vi "Dashboard Main.vi"() -> ()   [LabVIEW 2012]
uses:
  <vilib>/event_ctls.llb/eventvkey.ctl
  <vilib>/Rock Robotics/Network Tables/NT Read Name Cache.vi
  <vilib>/Rock Robotics/Network Tables/NT Globals.vi
  <vilib>/Rock Robotics/Network Tables/Field Data Manager.vi
  <vilib>/Rock Robotics/Network Tables/Table Manager.vi
  <vilib>/Rock Robotics/Network Tables/Report Read Error.vi
panel:
  out "Mode":enum8{"Tele-Op", "Auto", "Test", ""}(ring)=enum."Test"
  out "Camera IP":string
  out "JS1 Z":dbl(slide) scale=-1.0..1.0 scale format="%#_2e"
  out "JS2 Z":dbl(slide) scale=-1.0..1.0 scale format="%#_2e"
  out "Joystick 1":cluster{"X":dbl, "Y":dbl}[](graph)
  out "Joystick 2":cluster{"X":dbl, "Y":dbl}[](graph)
  out "JS Buttons 1":T1
  out "JS Buttons 2":T1
  out "MotorSlide4":dbl(slide) scale=-1.0..1.0 scale format="%#_2e"
  out "MotorSlide3":dbl(slide) scale=-1.0..1.0 scale format="%#_2e"
  out "MotorSlide2":dbl(slide) scale=-1.0..1.0 scale format="%#_2e"
  in  "MotorName3":string="Front Left"
  in  "MotorName4":string="Front Right"
  in  "MotorName1":string="Rear Left"
  in  "MotorName2":string="Rear Right"
  out "MotorChart4":dbl(graph)
  out "MotorChart3":dbl(graph)
  out "MotorChart2":dbl(graph)
  out "MotorSlide1":dbl(slide) scale=-1.0..1.0 scale format="%#_2e"
  out "MotorChart1":dbl(graph)
  out "Battery Value":dbl(slide) scale=0.0..14.0 scale format="%#_2e"
  out "Robot IP":string
  out "Battery":sgl(graph)
  in  "Dashboard Tab":enum32{"Operation", "Test", "Checklist"}(tab)
  out "Motor 0":dbl
  out "Motor 4":dbl
  out "Motor 3":dbl
  out "Motor 2":dbl
  out "Motor 1":dbl
  out "Y Axis":dbl
  out "X Axis":dbl
  in  "Checkbox 2":bool
  in  "Checkbox 1":bool
  in  "Slider 1":dbl(slide) scale=0.0..100.0
  in  "ServoValue":dbl(slide) scale=0.0..170.0 scale format="%#_3g"
  in  "On/Off":bool caption="Solenoid"
  in  "Test Name":u16(ring) items=["Select the test to run...", "Example Test", "", "Tests are read from", "Public\\Documents\\FRC\\Tests.txt", "", "Modify file to customize list."]
  in  "Test Tree":string(tree)
  in  "Motor":cluster{"Value":dbl, "Enable":bool} {"Value" scale=-1.0..1.0 scale format="%#_3g"}
  out "Progress":T2 {"Test Progress" scale=0.0..100.0}
  in  "Rev/Fwd":cluster{"Forward":bool, "Reverse":bool}
  in  "Listbox":i32(listbox)
  in  "Viewer":T3(tab)
  out "Image Error Message":string="Timeout in Camera Communications"
  in  "Video Enable":bool=TRUE
  out "Camera Image":T4(plugin-control)
  out "Buttons 1":cluster{"1":bool, "2":bool, "3":bool}
  out "Kinect 1":cluster{"X":dbl, "Y":dbl, "Z":dbl} {"X" scale=1.0..-1.0; "Y" scale=1.0..-1.0; "Z" scale=1.0..-1.0}
  out "Buttons 2":cluster{"1":bool, "2":bool, "3":bool}
  out "Kinect 2":cluster{"X":dbl, "Y":dbl, "Z":dbl} {"X" scale=1.0..-1.0; "Y" scale=1.0..-1.0; "Z" scale=1.0..-1.0}
  out "Version":string
  out "Skeleton Picture":picture
  out "Players":i8
  out "Tree":string(tree)
  # "Drive & Motors"
  # "Robot IP:"
  # "Customize by placing controls and indicators here and name to match\nDashboard Variables on robot."
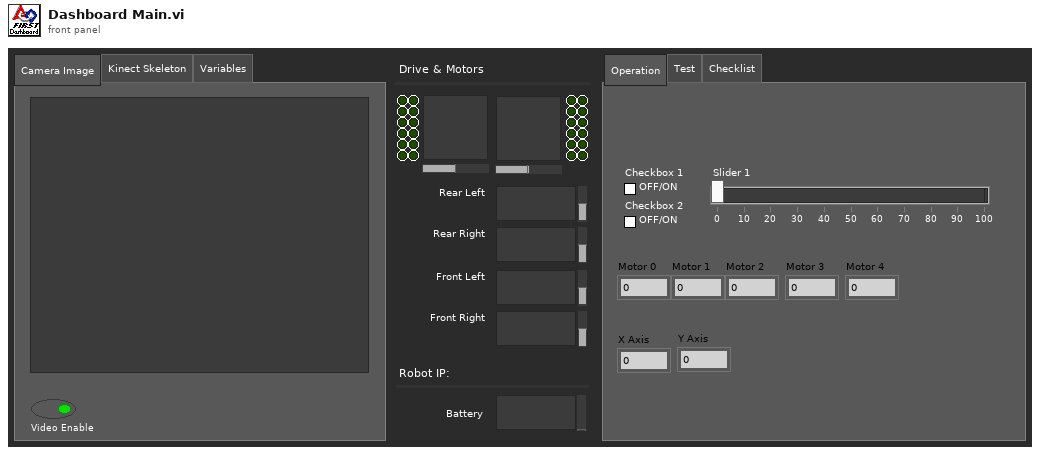
[diagram p1: front panel]
types:
  T1 = cluster{bool, bool, bool, bool, bool, bool, bool, bool, bool, bool, bool, bool}
  T2 = cluster{"Test Progress":u8, "Test Progress Text":string}
  T3 = enum32{"Camera Image", "Kinect Skeleton", "Variables"}
  T4 = typedef "IMAQ Image.ctl" = refnum<image>
  T5 = typedef "Image Type" = u32
  T6 = typedef "SkeletonTrackState.ctl" = enum32{"NotTracked", "PositionOnly", "Tracked"}
  T7 = cluster{"TrackingState":u8[], "Position":cluster{"x":sgl, "y":sgl, "z":sgl}, cluster{"x":sgl, "y":sgl, "z":sgl, sgl}[], "TrackState":T6}
  T8 = cluster{cluster{"ScaledToPercentRange":dbl, "ScaledToPercentRange":dbl, "ScaledToPercentRange":dbl}, cluster{bool, bool, bool}}[]
  T9 = typedef "LVBoundsTypeDef.ctl" = cluster{"Width":u32, "Height":u32}
  T10 = cluster{cluster{"ScaledToPercentRange":dbl, "ScaledToPercentRange":dbl, "ScaledToPercentRange":dbl}, cluster{bool, bool, bool}}
  T11 = cluster{"ScaledToPercentRange":dbl, "ScaledToPercentRange":dbl, "ScaledToPercentRange":dbl}
  T12 = typedef "LVRectTypeDef.ctl" = cluster{"Left":i16, "Top":i16, "Right":i16, "Bottom":i16}
  T13 = cluster{"Competition mode":bool, "Robot Link":bool, "Autonomous":bool, "Enabled":bool, "E-Stop":bool, "Simulated":bool, "TestMode":bool, "Docked Window":bool}
  T14 = cluster{"Boolean Array[0]":bool, "Boolean Array[1]":bool, "Boolean Array[2]":bool, "Boolean Array[3]":bool, "Boolean Array[4]":bool, "Boolean Array[5]":bool, "Boolean Array[6]":bool, "Boolean Array[7]":bool, "Boolean Array[8]":bool, "Boolean Array[9]":bool, "Boolean Array[10]":bool, "Boolean Array[11]":bool}
  T15 = typedef "eventvkey.ctl" = enum16{"ASCII", "Enter", "Return", "Shift", "Ctrl", "Alt", "Cmd", "Opt", "Caps", "NumLock", "Clear", "Break", "Up", "Down", "Left", "Right", "Insert", "Delete", "Home", "End", "PageUp", "PageDown", "Escape", "Help", "Pause", "ScrollLock", "F1", "F2", "F3", "F4", "F5", "F6", "F7", "F8", "F9", "F10", "F11", "F12", "F13", "F14", "F15", "F16", "F17", "F18", "F19", "F20", "F21", "F22", "F23", "F24", "Play", "VolumeUp", "VolumeDown", "Mute", "Two Byte Char"}
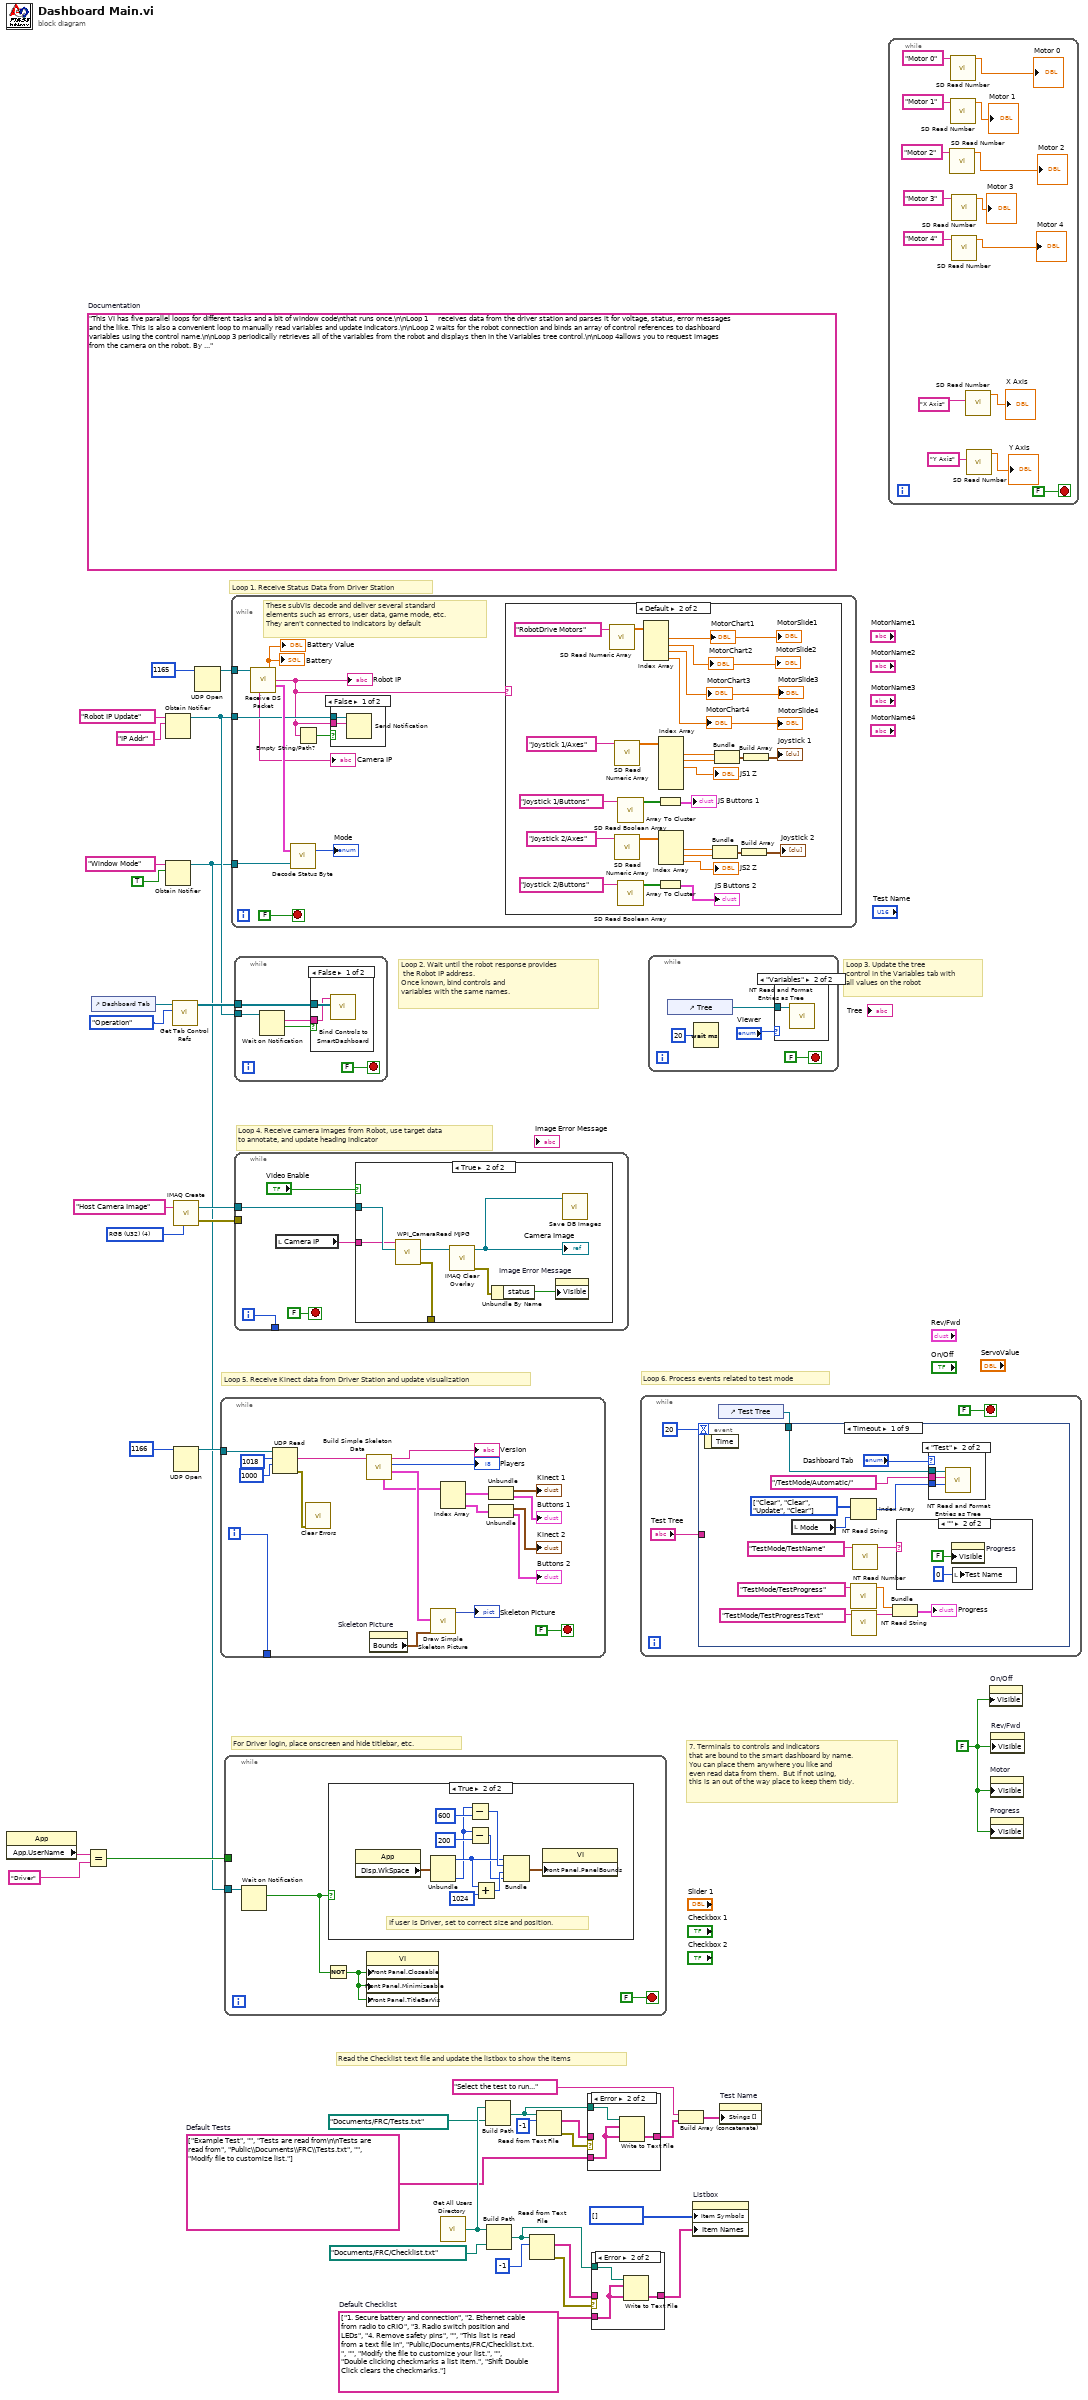
[diagram p0: block diagram]
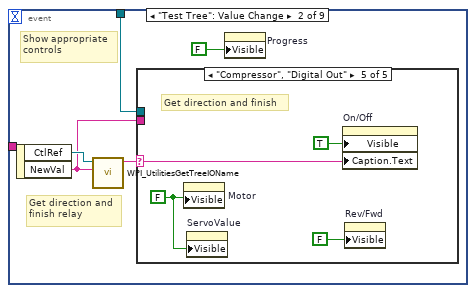
[diagram p7: hidden frame]
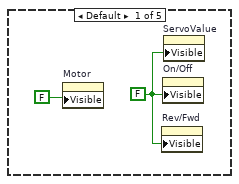
[diagram p8: hidden frame]
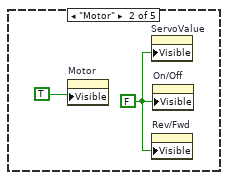
[diagram p9: hidden frame]
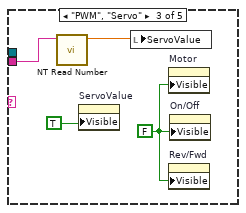
[diagram p10: hidden frame]
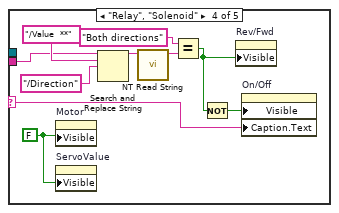
[diagram p11: hidden frame]
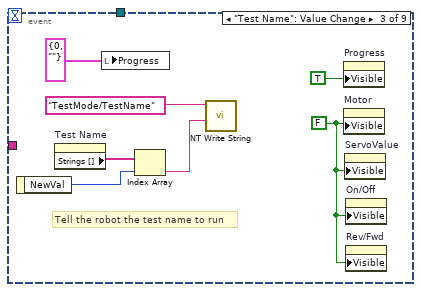
[diagram p12: hidden frame]
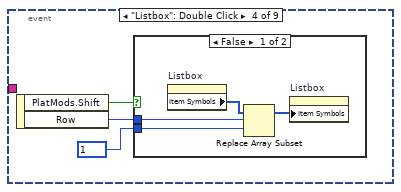
[diagram p13: hidden frame]
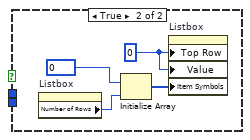
[diagram p14: hidden frame]
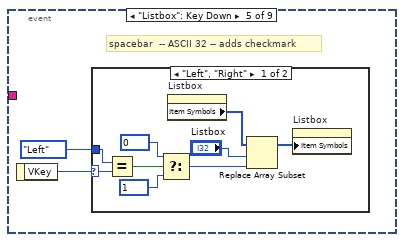
[diagram p15: hidden frame]
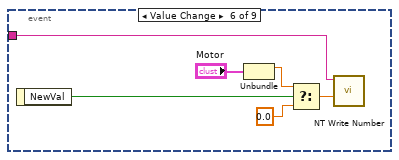
[diagram p17: hidden frame]
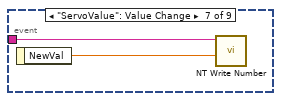
[diagram p18: hidden frame]
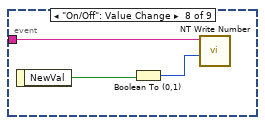
[diagram p19: hidden frame]
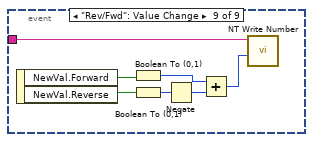
[diagram p20: hidden frame]
diagram:
  w3 = string[] ["1. Secure battery and connection", "2. Ethernet cable from radio to cRIO", "3. Radio switch position and LEDs", "4. Remove safety pins", "", "This list is read from a text file in", "Public/Documents/FRC/Checklist.txt.", "", "Modify the file to customize your list.", "", "Double clicking checkmarks a list item.", "Shift Double Click clears the checkmarks."]  # Default Checklist
  w8 = string[] ["Example Test", "", "Tests are read from\n\nTests are read from", "Public\\Documents\\FRC\\Tests.txt", "", "Modify file to customize list."]  # Default Tests
  w1 = FALSE ("Visible")
  (unwired) "This VI has five parallel loops for different tasks and a bit of window code\nthat runs once.\n\nLoop 1     receives data from the driver station and parses it for voltage, status, error messages and the like. This is also a convenient loop to manually read variables and update indicators.\n\nLoop 2 waits for the robot connection and binds an array of control references to dashboard variables using the control name.\n\nLoop 3 periodically retrieves all of the variables from the robot and displays then in the Variables tree control.\n\nLoop 4allows you to request images from the camera on the robot. By default, it reads the images using MJPG stream, but has compatibility for the older setup which used JPGs.\n\nLoop 5 processes any data from the Kinect server and shows the skeleton and Kinect stick values in the Kinect tab.\n\nLoop 6 process events for the TestMode tree, listbox, ring, and actuator\n\nLoop 7 calculates and updates the window location, size, and style. The checklist and tests are loaded from text files and placed into the controls.\n\nAdding new indicators or controls:\nAdd them to the panel in the Operations tab and name them the same as the SmartDashboard variable on the robot. The binding loop will keep them synchronized."  # Documentation
  w37 = T5 4 items=["Grayscale (U8)", "Grayscale (I16)", "Grayscale (SGL)", "Complex (CSG)", "RGB (U32)", "HSL (U32)", "RGB (U64)"] ("Image Type")
  # "Loop 6. Process events related to test mode"
  # "Read the Checklist text file and update the listbox to show the items"
  # "7. Terminals to controls and indicators\nthat are bound to the smart dashboard by name.\nYou can place them anywhere you like and\neven read data from them.  But if not using,\nthis is an out of the way place to keep them tidy."
  # "Loop 3. Update the tree\ncontrol in the Variables tab with\nall values on the robot"
  # "Loop 2. Wait until the robot response provides\n the Robot IP address.\nOnce known, bind controls and\nvariables with the same names."
  # "Loop 5. Receive Kinect data from Driver Station and update visualization"
  # "For Driver login, place onscreen and hide titlebar, etc."
  # "Loop 1. Receive Status Data from Driver Station"
  # "Loop 4. Receive camera images from Robot, use target data\nto annotate, and update heading indicator"
  n1 = property class="App"() -> ("App.UserName"=w32:string)  [unwired: 2 in, 2 out]
  n2 = Equal?(x=w32, y="Driver") -> (x = y?=w31:bool)
  n3 = control-ref of="Dashboard Tab"() -> (w27:refnum<vi>)
  n4 = Obtain Notifier(name (unnamed)="Robot IP Update", notification data type="IP Addr" ("name (unnamed)")) -> (notifier out=w24:refnum<notifier>)  [unwired: 2 in, 2 out]
  n5 = Obtain Notifier(name (unnamed)="Window Mode", notification data type=TRUE) -> (notifier out=w12:refnum<notifier>)  [unwired: 2 in, 2 out]
  n6 = call <vilib>:"Get Tab Control Refs.vi"("Page Index"=enum32{"Operation", "Test"}."Operation" ("Dashboard Tab"), "TabControl in"=w27) -> ("ControlsOnPage"=w28:refnum<vi>[])  [unwired: 9 in]
  n7 = call "IMAQ Create"("Image Name"="Host Camera Image", "Image Type"=w37) -> ("New Image"=w35:T4, "error out"=w34:errorcluster)  [unwired: 2 in, 1 out]
  n8 = UDP Open(11:u16 1166 ("port")) -> (port=w29:refnum<k16>)  [unwired: 2 in, 4 out]
  n9 = UDP Open(11:u16 1165 ("port")) -> (port=w38:refnum<k16>)  [unwired: 2 in, 4 out]
  n10 = while {
    tunnel: w29 -> [w56]
    tunnel: [w40] -> _
    i -> [w40]
    stop <- FALSE stop-if-true
    n11 = UDP Read(connection ID=w56, max size (548)=1018 ("bytes to read"), timeout ms (25000)=1000) -> (data out=w50:string, error out=w48:errorcluster)  [unwired: 1 in, 3 out]
    n12 = call <vilib>:"Clear Errors.vi"("error in (no error)"=w48) -> ()  [unwired: 6 in, 1 out]
    n13 = call "Build Simple Skeleton Data.vi"("data out"=w50) -> ("Skeleton Data"=w51:T7, "NumPlayers"=→"Players":i8, "Version String"=→"Version":string, "Simple Joystick Info"=w47:T8)  [unwired: 6 in, 1 out]
    n14 = property on="Skeleton Picture" class="Pict"() -> ("Bounds"=w52:T9)  [unwired: 2 in, 2 out]
    n15 = call "Draw Simple Skeleton Picture.vi"("Bounds"=w52, "Simple Skeleton"=w51) -> ("new picture out"=→"Skeleton Picture":picture)  [unwired: 9 in]
    n16 = Index Array(array=w47) -> (element #1=w46:T10, element #2=w45:T10)  [unwired: 2 in]
    n17 = Unbundle(w46) -> (→"Kinect 1":T11, →"Buttons 1":cluster{bool, bool, bool})
    n18 = Unbundle(w45) -> (→"Kinect 2":T11, →"Buttons 2":cluster{bool, bool, bool})
  }
  n19 = while {
    tunnel: w31 -> [_]
    tunnel: w12 -> [w61]
    stop <- FALSE stop-if-true
    n20 = Wait on Notification(notifier=w61) -> (notification=w59:bool)  [unwired: 3 in, 3 out]
    n21 = Not(x=w59) -> (.not. x?=w60:bool)
    n22 = case shown="True" w59 {
      frame False {
      }
      frame True {
        # "If user is Driver, set to correct size and position."
        n23 = property class="App"() -> ("Disp.WkSpace"=w72:T12)  [unwired: 2 in, 2 out]
        n24 = Unbundle(w72) -> ("Left"=w67:i16, "Bottom"=w63:i16)  [unwired: 2 out]
        n25 = Subtract(x=w63, y=600) -> (x-y=w69:i32)
        n26 = Subtract(x=w63, y=200) -> (x-y=w64:i32)
        n27 = Add(x=w67, y=1024) -> (x+y=w68:i32)
        n28 = Bundle("Left"=w67, w69, w68, w64) -> (w71:cluster{"Left":i16, i32, i32, i32})  [unwired: 1 out]
        n29 = property class="VI"("Front Panel.PanelBounds"=w71) -> ()  [unwired: 2 in, 2 out]
      }
    }
    n30 = property class="VI"("Front Panel.Closeable"=w60, "Front Panel.Minimizeable"=w60, "Front Panel.TitleBarVis"=w60) -> ()  [unwired: 2 in, 2 out]
  }
  n31 = while {
    tunnel: w38 -> [w80]
    tunnel: w24 -> [w78]
    tunnel: w12 -> [w75]
    stop <- FALSE stop-if-true
    # "These subVIs decode and deliver several standard\nelements such as errors, user data, game mode, etc.\nThey aren't connected to indicators by default"
    n32 = call "Receive DS Packet.vi"("Recv Socket"=w80) -> ("Battery"=→"Battery" →"Battery Value":sgl, "Robot IP Address"=w77:string, "Status"=w81:T13, "Camera IP Address"=→"Camera IP":string)  [unwired: 1 in, 10 out]
    "Robot IP" <- w77
    n33 = call "Decode Status Byte.vi"("Window Mode Notifier"=w75, "Status"=w81) -> ("Mode"=→"Mode":enum8{"Tele-Op", "Auto", "Test", ""})  [unwired: 1 out]
    n34 = Empty String/Path?(string/path=w77) -> (empty?=w76:bool)
    n35 = case shown="False" w76 {
      tunnel: w78 -> [w110 _]
      tunnel: w77 -> [w109 _]
      frame False {
        n36 = Send Notification(notification=w109, notifier=w110) -> ()  [unwired: 1 in, 2 out]
      }
      frame True {
      }
    }
    n37 = case shown="Default" w77 {
      frame "" {
        # "Robot not responding, don't poll the variables"
      }
      frame Default {
        n38 = call <vilib>:"SD Read Numeric Array.vi"("Name"="RobotDrive Motors") -> ("Numeric Array"=w105:dbl[])  [unwired: 8 in, 2 out]
        n39 = call <vilib>:"SD Read Numeric Array.vi"("Name"="Joystick 1/Axes") -> ("Numeric Array"=w98:dbl[])  [unwired: 8 in, 2 out]
        n40 = call <vilib>:"SD Read Numeric Array.vi"("Name"="Joystick 2/Axes") -> ("Numeric Array"=w92:dbl[])  [unwired: 8 in, 2 out]
        n41 = call <vilib>:"SD Read Boolean Array.vi"("Name"="Joystick 1/Buttons") -> ("Boolean Array"=w100:bool[])  [unwired: 8 in, 2 out]
        n42 = call <vilib>:"SD Read Boolean Array.vi"("Name"="Joystick 2/Buttons") -> ("Boolean Array"=w91:bool[])  [unwired: 8 in, 2 out]
        n43 = Index Array(array=w105) -> (element #1=→"MotorChart1" →"MotorSlide1":dbl, element #2=→"MotorSlide2" →"MotorChart2":dbl, element #3=→"MotorChart3" →"MotorSlide3":dbl, element #4=→"MotorChart4" →"MotorSlide4":dbl)  [unwired: 4 in]
        n44 = Array To Cluster(array=w100) -> (cluster=→"JS Buttons 1":T14)
        n45 = Array To Cluster(array=w91) -> (cluster=→"JS Buttons 2":T14)
        n46 = Index Array(array=w98) -> (element #1=w95:dbl, element #2=w96:dbl, element #3=→"JS1 Z":dbl)  [unwired: 6 in, 3 out]
        n47 = Index Array(array=w92) -> (element #1=w87:dbl, element #2=w86:dbl, element #3=→"JS2 Z":dbl)  [unwired: 3 in]
        n48 = Bundle("Numeric"=w87, "Numeric"=w86) -> (w88:cluster{"Numeric":dbl, "Numeric":dbl})  [unwired: 1 in]
        n49 = Bundle("Numeric"=w95, "Numeric"=w96) -> (w94:cluster{"Numeric":dbl, "Numeric":dbl})  [unwired: 1 in]
        n50 = Build Array(w88) -> (→"Joystick 2":cluster{"Numeric":dbl, "Numeric":dbl}[])
        n51 = Build Array(w94) -> (→"Joystick 1":cluster{"Numeric":dbl, "Numeric":dbl}[])
      }
    }
  }
  n52 = while {
    tunnel: w28 -> [w115]
    tunnel: w24 -> [w112]
    stop <- FALSE stop-if-true
    n53 = Wait on Notification(notifier=w112) -> (notification=w111:string, timed out?=w113:bool)  [unwired: 3 in, 2 out]
    n54 = case shown="False" w113 {
      tunnel: w115 -> [w117 _]
      tunnel: w111 -> [w116 _]
      frame False {
        n55 = call <vilib>:"Bind Controls to SmartDashboard.vi"("Bound Control Refs"=w117, "Server IP Address"=w116) -> ()  [unwired: 10 in]
      }
      frame True {
      }
    }
  }
  n56 = while {
    tunnel: w35 -> [w121]
    tunnel: w34 -> [_]
    tunnel: [w119] -> _
    i -> [w119]
    stop <- FALSE stop-if-true
    n57 = local read "Camera IP"() -> (w118:string)
    n58 = case shown="True" "Video Enable" {
      tunnel: w118 -> [w125 w127]
      tunnel: w121 -> [w124 w133]
      tunnel: [_ w128] -> _
      frame False {
        # "Sleep for 500ms"
        n59 = call <vilib>:"WPI_CameraRead MJPG.vi"("Operation"=enum16{"Read", "Reopen", "Close"}."Close", "Image"=w124, "address"=w125) -> ()  [unwired: 7 in, 2 out]
        n60 = Wait Until Next ms Multiple(millisecond multiple=u32 500) -> ()  [unwired: 1 out]
      }
      frame True {
        n61 = call <vilib>:"WPI_CameraRead MJPG.vi"("Image"=w133, "address"=w127) -> ("error out"=w128:errorcluster, "Image Out"=w130:T4)  [unwired: 8 in]
        n62 = call "IMAQ Clear Overlay"("Image"=w130) -> ("error out"=w131:errorcluster, "Image Out"=w129:T4)  [unwired: 2 in, 7 out]
        "Camera Image" <- w129
        n63 = Unbundle By Name(w131) -> ("status"=w132:bool)
        n64 = property on="Image Error Message" class="Str"("Visible"=w132) -> ()  [unwired: 2 in, 2 out]
        n65 = call "Save DB Images.vi"("Image"=w129) -> ()  [unwired: 2 in, 1 out]
      }
    }
  }
  n66 = call "Get All Users Directory.vi"() -> ("All User Path"=w19:path)
  n67 = Build Path(base path=w19, name or relative path=path "Documents/FRC/Tests.txt") -> (appended path=w7:path)
  n68 = Build Path(base path=w19, name or relative path=path "Documents/FRC/Checklist.txt") -> (appended path=w4:path)
  n69 = Read from Text File(file (use dialog)=w4, count=-1 ("timeout ms (25000)")) -> (text=w5:string[], error out=w6:errorcluster)  [unwired: 2 in, 2 out]
  n70 = Read from Text File(file (use dialog)=w7, count=-1 ("timeout ms (25000)")) -> (text=w10:string[], error out=w11:errorcluster)  [unwired: 2 in, 2 out]
  n71 = case shown="Error" w11 {
    tunnel: w10 -> [w134 _]
    tunnel: [w134 w135] -> w9
    tunnel: w8 -> [_ w135]
    tunnel: w7 -> [_ w136]
    frame No Error {
    }
    frame Error {
      n72 = Write to Text File(file (use dialog)=w136, text=w135) -> ()  [unwired: 2 in, 3 out]
    }
  }
  n73 = case shown="Error" w6 {
    tunnel: w5 -> [w137 _]
    tunnel: [w137 w138] -> w2
    tunnel: w3 -> [_ w138]
    tunnel: w4 -> [_ w139]
    frame No Error {
    }
    frame Error {
      n74 = Write to Text File(file (use dialog)=w139, text=w138) -> ()  [unwired: 2 in, 3 out]
    }
  }
  n75 = while {
    stop <- FALSE stop-if-true
    n76 = control-ref of="Test Tree"() -> (w141:refnum<vi>)
    n77 = event shown="[0] Timeout" {
      selector: _ -> [_ _ _ _ _ _ _ _ _]
      dyn-events: _ -> [_ _ _ _ _ _ _ _ _]
      timeout: u32 20 ("milliseconds to wait") -> [_ _ _ _ _ _ _ _ _]
      tunnel: w141 -> [w152 w163 _ _ _ _ _ _ _]
      tunnel: "Test Tree" -> [_ _ _ _ _ w218 w225 w226 w229]
      event Timeout {
        w145 = enum16{"Update", "Clear"}[] [enum."Clear", enum."Clear", enum."Update", enum."Clear"] items=["Update", "Clear"]
        n78 = event-data() -> ()  [unwired: 1 in, 1 out]
        n79 = local read "Mode"() -> (w146:enum8{"Tele-Op", "Auto", "Test", ""})
        n80 = Index Array(array=w145, index=w146) -> (element=w144:enum16{"Update", "Clear"})
        n81 = call <vilib>:"NT Read Number.vi"("Name"="TestMode/TestProgress") -> ("Numeric"=w149:dbl)  [unwired: 9 in, 1 out]
        n82 = call <vilib>:"NT Read String.vi"("Name"="TestMode/TestProgressText") -> ("String"=w148:string)  [unwired: 9 in, 1 out]
        n83 = call <vilib>:"NT Read String.vi"("Name"="TestMode/TestName") -> ("String"=w155:string)  [unwired: 9 in, 1 out]
        n84 = Bundle("Numeric"=w149, "String"=w148) -> (→"Progress":cluster{"Numeric":dbl, "String":string})  [unwired: 1 in]
        n85 = case shown="\"\"" w155 {
          frame Default {
          }
          frame "" {
            n86 = property on="Progress" class="Clust (strict)"("Visible"=FALSE) -> ()  [unwired: 2 in, 2 out]
            n87 = local write "Test Name"(u16 0) -> ()
          }
        }
        n88 = case shown="\"Test\"" "Dashboard Tab" {
          tunnel: w152 -> [_ w159]
          tunnel: "/TestMode/Automatic/" ("Name Pattern") -> [_ w158]
          tunnel: w144 -> [_ w157]
          frame "Operation", Default {
          }
          frame "Test" {
            n89 = call <vilib>:"NT Read and Format Entries as Tree.vi"("Operation"=w157, "Name Pattern"=w158, "Tree Refnum"=w159) -> ()  [unwired: 7 in, 2 out]
          }
        }
      }
      event "Test Tree": Value Change {
        # "Get direction and\nfinish relay"
        # "Show appropriate\ncontrols"
        n90 = event-data() -> ("CtlRef"=w165:refnum<vi>, "NewVal"=w162:string)  [unwired: 1 in]
        n91 = call <vilib>:"WPI_UtilitiesGetTreeIOName.vi"("NewVal"=w162, "TreeControl in"=w165) -> ("I/O Name"=w166:string)  [unwired: 9 in]
        n92 = case shown="\"Compressor\", \"Digital Out\"" w166 {
          selector: w166 -> [_ _ _ w176 w185]
          tunnel: w163 -> [_ _ _ _ _]
          tunnel: w162 -> [_ _ w172 w175 _]
          frame Default {
            w167 = FALSE ("Visible")
            n93 = property on="Motor" class="Clust (strict)"("Visible"=FALSE) -> ()  [unwired: 2 in, 2 out]
            n94 = property on="Rev/Fwd" class="Clust (strict)"("Visible"=w167) -> ()  [unwired: 2 in, 2 out]
            n95 = property on="On/Off" class="Bool (strict)"("Visible"=w167) -> ()  [unwired: 2 in, 2 out]
            n96 = property on="ServoValue" class="Slide (strict)"("Visible"=w167) -> ()  [unwired: 2 in, 2 out]
          }
          frame "Motor" {
            w169 = FALSE ("Visible")
            n97 = property on="Motor" class="Clust (strict)"("Visible"=TRUE) -> ()  [unwired: 2 in, 2 out]
            n98 = property on="ServoValue" class="Slide (strict)"("Visible"=w169) -> ()  [unwired: 2 in, 2 out]
            n99 = property on="Rev/Fwd" class="Clust (strict)"("Visible"=w169) -> ()  [unwired: 2 in, 2 out]
            n100 = property on="On/Off" class="Bool (strict)"("Visible"=w169) -> ()  [unwired: 2 in, 2 out]
          }
          frame "PWM", "Servo" {
            w174 = FALSE ("Visible")
            n101 = call <vilib>:"NT Read Number.vi"("Name"=w172) -> ("Numeric"=w171:dbl)  [unwired: 9 in, 1 out]
            n102 = property on="ServoValue" class="Slide (strict)"("Visible"=TRUE) -> ()  [unwired: 2 in, 2 out]
            n103 = local write "ServoValue"(w171) -> ()
            n104 = property on="Motor" class="Clust (strict)"("Visible"=w174) -> ()  [unwired: 2 in, 2 out]
            n105 = property on="Rev/Fwd" class="Clust (strict)"("Visible"=w174) -> ()  [unwired: 2 in, 2 out]
            n106 = property on="On/Off" class="Bool (strict)"("Visible"=w174) -> ()  [unwired: 2 in, 2 out]
          }
          frame "Relay", "Solenoid" {
            w177 = FALSE ("Visible")
            n107 = property on="Motor" class="Clust (strict)"("Visible"=w177) -> ()  [unwired: 2 in, 2 out]
            n108 = property on="ServoValue" class="Slide (strict)"("Visible"=w177) -> ()  [unwired: 2 in, 2 out]
            n109 = Search and Replace String(input string=w175, search string="/Value  **", replace string="/Direction") -> (result string=w182:string)  [unwired: 5 in, 3 out]
            n110 = call <vilib>:"NT Read String.vi"("Name"=w182) -> ("String"=w180:string)  [unwired: 9 in, 1 out]
            n111 = Equal?(x="Both directions", y=w180) -> (x = y?=w178:bool)
            n112 = Not(x=w178) -> (.not. x?=w179:bool)
            n113 = property on="Rev/Fwd" class="Clust (strict)"("Visible"=w178) -> ()  [unwired: 2 in, 2 out]
            n114 = property on="On/Off" class="Bool (strict)"("Visible"=w179, "Caption.Text"=w176) -> ()  [unwired: 2 in, 2 out]
          }
          frame "Compressor", "Digital Out" {
            w187 = FALSE ("Visible")
            # "Get direction and finish"
            n115 = property on="Motor" class="Clust (strict)"("Visible"=w187) -> ()  [unwired: 2 in, 2 out]
            n116 = property on="ServoValue" class="Slide (strict)"("Visible"=w187) -> ()  [unwired: 2 in, 2 out]
            n117 = property on="On/Off" class="Bool (strict)"("Visible"=TRUE, "Caption.Text"=w185) -> ()  [unwired: 2 in, 2 out]
            n118 = property on="Rev/Fwd" class="Clust (strict)"("Visible"=FALSE) -> ()  [unwired: 2 in, 2 out]
          }
        }
        n119 = property on="Progress" class="Clust (strict)"("Visible"=FALSE) -> ()  [unwired: 2 in, 2 out]
      }
      event "Test Name": Value Change {
        w189 = FALSE ("Visible")
        # "Tell the robot the test name to run"
        n120 = event-data() -> ("NewVal"=w193:u16)  [unwired: 1 in]
        n121 = property on="Test Name" class="Ring (strict)"() -> ("Strings []"=w194:string[])  [unwired: 2 in, 2 out]
        n122 = local write "Progress"(T2 {"Test Progress"=0, "Test Progress Text"=""} ("Progress")) -> ()
        n123 = Index Array(array=w194, index=w193) -> (element=w192:string)
        n124 = call <vilib>:"NT Write String.vi"("String"=w192, "Name"="TestMode/TestName") -> ()  [unwired: 9 in, 1 out]
        n125 = property on="Progress" class="Clust (strict)"("Visible"=TRUE) -> ()  [unwired: 2 in, 2 out]
        n126 = property on="Motor" class="Clust (strict)"("Visible"=w189) -> ()  [unwired: 2 in, 2 out]
        n127 = property on="ServoValue" class="Slide (strict)"("Visible"=w189) -> ()  [unwired: 2 in, 2 out]
        n128 = property on="On/Off" class="Bool (strict)"("Visible"=w189) -> ()  [unwired: 2 in, 2 out]
        n129 = property on="Rev/Fwd" class="Clust (strict)"("Visible"=w189) -> ()  [unwired: 2 in, 2 out]
      }
      event "Listbox": Double Click {
        n130 = event-data() -> ("PlatMods.Shift"=w196:bool, "Row"=w198:i32)  [unwired: 1 in]
        n131 = case shown="False" w196 {
          tunnel: w198 -> [w202 _]
          tunnel: 1 -> [w201 _]
          frame False {
            n132 = property on="Listbox" class="LstBox (strict)"() -> ("Item Symbols"=w200:i32[])  [unwired: 2 in, 2 out]
            n133 = Replace Array Subset(array=w200, new element=w201, index=w202) -> (w199:i32[])
            n134 = property on="Listbox" class="LstBox (strict)"("Item Symbols"=w199) -> ()  [unwired: 2 in, 2 out]
          }
          frame True {
            w203 = 0 ("Top Row")
            n135 = property on="Listbox" class="LstBox (strict)"() -> ("Number of Rows"=w205:u32)  [unwired: 2 in, 2 out]
            n136 = Initialize Array(0, w205) -> (w204:i32[])
            n137 = property on="Listbox" class="LstBox (strict)"("Top Row"=w203, "Value"=w203, "Item Symbols"=w204) -> ()  [unwired: 2 in, 2 out]
          }
        }
      }
      event "Listbox": Key Down {
        # "spacebar  -- ASCII 32 -- adds checkmark"
        n138 = event-data() -> ("VKey"=w208:T15)  [unwired: 1 in]
        n139 = case shown="\"Left\", \"Right\"" w208 {
          selector: w208 -> [w213 _]
          tunnel: eventvkey."Left" ("VKey") -> [w211 _]
          frame "Left", "Right" {
            n140 = Equal?(x=w211, y=w213) -> (x = y?=w212:bool)
            n141 = Select(t=0, s=w212, f=1) -> (s? t:f=w214:i32)
            n142 = property on="Listbox" class="LstBox (strict)"() -> ("Item Symbols"=w217:i32[])  [unwired: 2 in, 2 out]
            n143 = Replace Array Subset(array=w217, new element=w214, index="Listbox") -> (w216:i32[])
            n144 = property on="Listbox" class="LstBox (strict)"("Item Symbols"=w216) -> ()  [unwired: 2 in, 2 out]
          }
          frame Default {
          }
        }
      }
      event "Motor.Enable": Value Change {
        n145 = event-data() -> ("NewVal"=w222:bool)  [unwired: 1 in]
        n146 = Unbundle("Motor") -> ("Value"=w221:dbl)  [unwired: 1 out]
        n147 = Select(t=w221, s=w222, f=0.0) -> (s? t:f=w219:dbl)
        n148 = call <vilib>:"NT Write Number.vi"("Numeric"=w219, "Name"=w218) -> ()  [unwired: 9 in, 1 out]
      }
      event "ServoValue": Value Change {
        n149 = event-data() -> ("NewVal"=w224:dbl)  [unwired: 1 in]
        n150 = call <vilib>:"NT Write Number.vi"("Numeric"=w224, "Name"=w225) -> ()  [unwired: 9 in, 1 out]
      }
      event "On/Off": Value Change {
        n151 = event-data() -> ("NewVal"=w228:bool)  [unwired: 1 in]
        n152 = Boolean To (0,1)(Boolean=w228) -> (0, 1=w227:i16)
        n153 = call <vilib>:"NT Write Number.vi"("Numeric"=w227, "Name"=w226) -> ()  [unwired: 9 in, 1 out]
      }
      event "Rev/Fwd": Value Change {
        n154 = event-data() -> ("NewVal.Forward"=w235:bool, "NewVal.Reverse"=w234:bool)  [unwired: 1 in]
        n155 = Boolean To (0,1)(Boolean=w235) -> (0, 1=w231:i16)
        n156 = Boolean To (0,1)(Boolean=w234) -> (0, 1=w233:i16)
        n157 = Negate(x=w233) -> (-x=w232:i16)
        n158 = Add(x=w231, y=w232) -> (x+y=w230:i16)
        n159 = call <vilib>:"NT Write Number.vi"("Numeric"=w230, "Name"=w229) -> ()  [unwired: 9 in, 1 out]
      }
    }
  }
  n160 = while {
    stop <- FALSE stop-if-true
    n161 = control-ref of="Tree"() -> (w237:refnum<vi>)
    n162 = Wait (ms)(milliseconds to wait=u32 20) -> ()  [unwired: 1 out]
    n163 = case shown="\"Variables\"" "Viewer" {
      tunnel: w237 -> [_ w240]
      frame "Camera Image", Default {
      }
      frame "Variables" {
        n164 = call <vilib>:"NT Read and Format Entries as Tree.vi"("Tree Refnum"=w240) -> ()  [unwired: 9 in, 2 out]
      }
    }
  }
  n165 = Build Array (concatenate)("Select the test to run...", w9) -> (w15:string[])
  n166 = property on="Listbox" class="LstBox (strict)"("Item Symbols"=i32[] [], "Item Names"=w2) -> ()  [unwired: 2 in, 2 out]
  n167 = property on="Test Name" class="Ring (strict)"("Strings []"=w15) -> ()  [unwired: 2 in, 2 out]
  n168 = while {
    stop <- FALSE stop-if-true
    n169 = call <vilib>:"SD Read Number.vi"("Name"="Motor 2") -> ("Numeric"=→"Motor 2":dbl)  [unwired: 8 in, 2 out]
    n170 = call <vilib>:"SD Read Number.vi"("Name"="Motor 0") -> ("Numeric"=→"Motor 0":dbl)  [unwired: 8 in, 2 out]
    n171 = call <vilib>:"SD Read Number.vi"("Name"="Motor 1") -> ("Numeric"=→"Motor 1":dbl)  [unwired: 8 in, 2 out]
    n172 = call <vilib>:"SD Read Number.vi"("Name"="Motor 3") -> ("Numeric"=→"Motor 3":dbl)  [unwired: 8 in, 2 out]
    n173 = call <vilib>:"SD Read Number.vi"("Name"="Motor 4") -> ("Numeric"=→"Motor 4":dbl)  [unwired: 8 in, 2 out]
    n174 = call <vilib>:"SD Read Number.vi"("Table Prefix"="X Axis") -> ("Numeric"=→"X Axis":dbl)  [unwired: 8 in, 2 out]
    n175 = call <vilib>:"SD Read Number.vi"("Table Prefix"="Y Axis") -> ("Numeric"=→"Y Axis":dbl)  [unwired: 8 in, 2 out]
  }
  n176 = property on="On/Off" class="Bool (strict)"("Visible"=w1) -> ()  [unwired: 2 in, 2 out]
  n177 = property on="Motor" class="Clust (strict)"("Visible"=w1) -> ()  [unwired: 2 in, 2 out]
  n178 = property on="Progress" class="Clust (strict)"("Visible"=w1) -> ()  [unwired: 2 in, 2 out]
  n179 = property on="Rev/Fwd" class="Clust (strict)"("Visible"=w1) -> ()  [unwired: 2 in, 2 out]
